vi "algoritmo_3 (1).vi"() -> ()   [LabVIEW 2024]
uses:
  <vilib>/Platform/TimedLoop/XDataNode/timing_clust.ctl
  <vilib>/Platform/TimedLoop/XDataNode/nitl_modes.ctl
  <vilib>/Platform/TimedLoop/XDataNode/wakeup.ctl
  <vilib>/MakerHub/LINX/Public/Peripherals/PWM/PWM Set Duty Cycle 1 Chan.vi
  <vilib>/MakerHub/LINX/Public/Utilities/Open Serial.vi
  <vilib>/MakerHub/LINX/Public/Peripherals/PWM/PWM Set Duty Cycle N Chans.vi
  <vilib>/platform/TimedLoop/XDataNode/XDataNode.xnode
  <vilib>/Platform/TimedLoop/XDataNode/XDNodeRunTimeDep.lvlib
  <vilib>/MakerHub/LINX/LMH-LINX.lvlib
  <vilib>/MakerHub/LINX/Public/Sensors/Distance/Ultrasonic/Ultrasonic.lvlib
  <vilib>/Analysis/NI_AALPro.lvlib
panel:
  in  "MODO":dbl
  in  "Estimacion":dbl(slide) scale=-41.0..41.0
  out "error":dbl
  out "POLO":dbl
  in  "Slide":dbl(slide) scale=-1.0..1.0
  out "PWM":dbl format="%0.2f"
  out "uk":dbl
  in  "Referencia":dbl(slide) scale=10.0..40.0
  out "ESTADO":dbl
  out "MINUTOS":dbl format="%#_2g"
  out "y_estimada":dbl
  out "error de estimacion":dbl
  out "THETA":cdb[](array[numeric])
  out "Waveform Chart":T1(graph)
  in  "stop":bool
  in  "Serial Port":refnum<visa-resource-name>="N/A"
  out "Error Out":errorcluster
  out "Y_Real":fxp<+/-,64,32>
  # "1 PARA CONTROLAR\n0 PARA ESTIMAR"
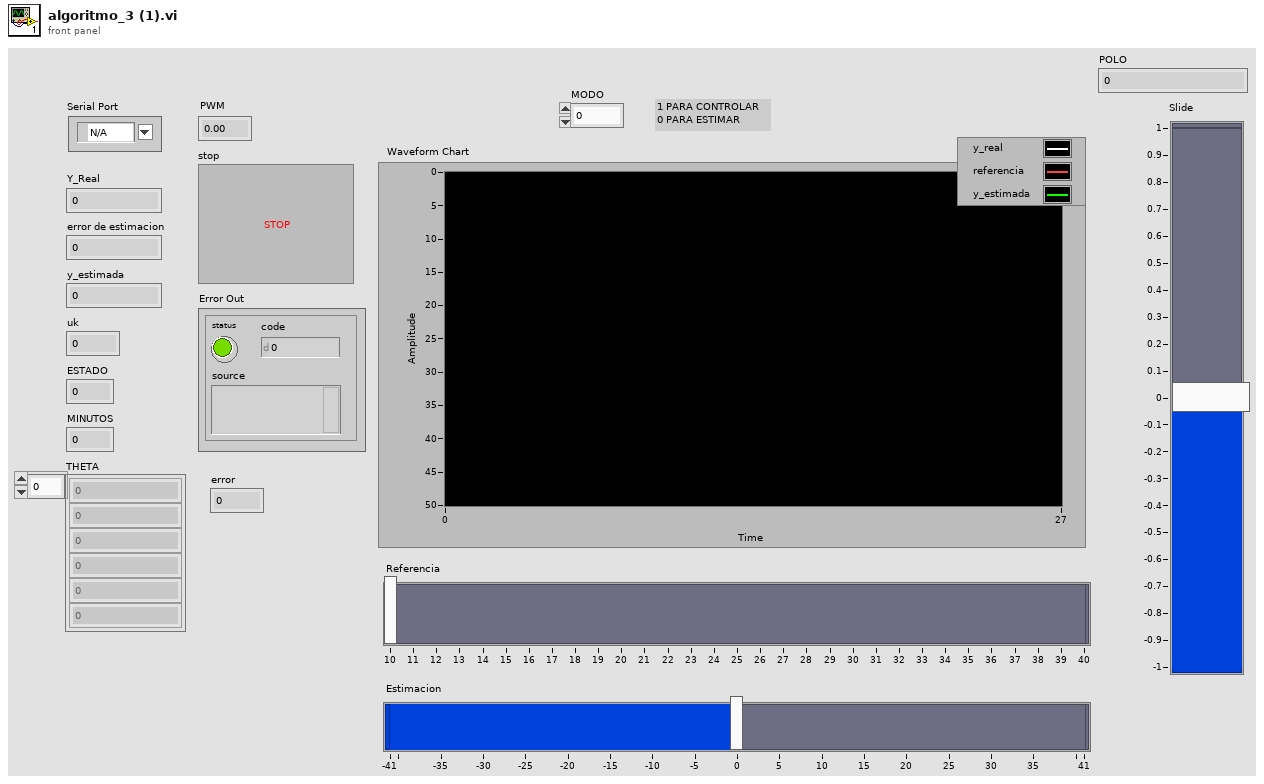
[diagram p1: front panel]
types:
  T1 = cluster{"Centimeters":dbl, "Referencia":dbl, dbl}
  T2 = typedef "LMH-LINX.lvlib/LINX Ref.ctl" = cluster{"IO":T3, "Interface":T4, "LINX Device Config":T5}
  T3 = typedef "LMH-LINX.lvlib/Platform.ctl" = enum16{"Remote", "Local"}
  T4 = typedef "LMH-LINX.lvlib/Interface.ctl" = enum16{"Serial", "TCP"}
  T5 = typedef "LMH-LINX.lvlib/Device.lvlib/LINX Device Config.ctl" = cluster{"Interface":T4, "COM Port":refnum<visa-resource-name>, "TCP Configuration":T6, "Device Family":u8, "Device ID":u8, "Device Name":string, "TCP Ref":refnum<k5>, "Channels":T7}
  T6 = typedef "LMH-LINX.lvlib/Device.lvlib/TCP Config.ctl" = cluster{"IP Address":string, "Port":u16}
  T7 = typedef "LMH-LINX.lvlib/Channels.ctl" = cluster{"DI":u8[], "DO":u8[], "AI":u8[], "AO":u8[], "PWM":u8[], "QE":u8[], "UART":u8[], "I2C 2":u8[], "SPI":u8[], "CAN":u8[], "Servo":u8[], "AI Ref (V)":dbl, "AI Resolution (Bits)":u8, "AO Ref (V)":dbl, "AO Resolution (Bits)":u8}
  T8 = typedef "XDNodeRunTimeDep.lvlib/timing_clust.ctl" = cluster{"Expected End [f-1]":u64, "Actual End [f-1]":u64, "Finished Late? [f-1]":bool, "Expected End [i-1]":u64, "Actual End [i-1]":u64, "Finished Late? [i-1]":bool, "Expected Start [i]":u64, "Actual Start [i]":u64, "Expected Start [f]":u64, "Actual Start [f]":u64, "Source Name":string, "Structure Name":string, "Period":i64, "Deadline":i64, "Offset":i64, "Start":i64, "Priority":i32, "Timeout":i32, "Mode":T9, "Wakeup Reason":T10, "Error":errorcluster, "Source Type":string, "Secondary Source Type":string, "Global End Time":u64, "Global Start Time":u64, "Frame Duration":u64, "Iteration Duration":u64, "Assigned CPU":i32, "I/O Scan Engine Mode":u32}
  T9 = typedef "XDNodeRunTimeDep.lvlib/nitl_modes.ctl" = enum32{"No Change", "Process missed periods, maintain original phase", "Discard missed periods, maintain original phase", "Process missed periods, ignore original phase", "Discard missed periods, ignore original phase"}
  T10 = typedef "XDNodeRunTimeDep.lvlib/wakeup.ctl" = enum32{"Normal", "Aborted", "Asynchronous wakeup", "Timing source error", "Timed loop error", "Timeout"}
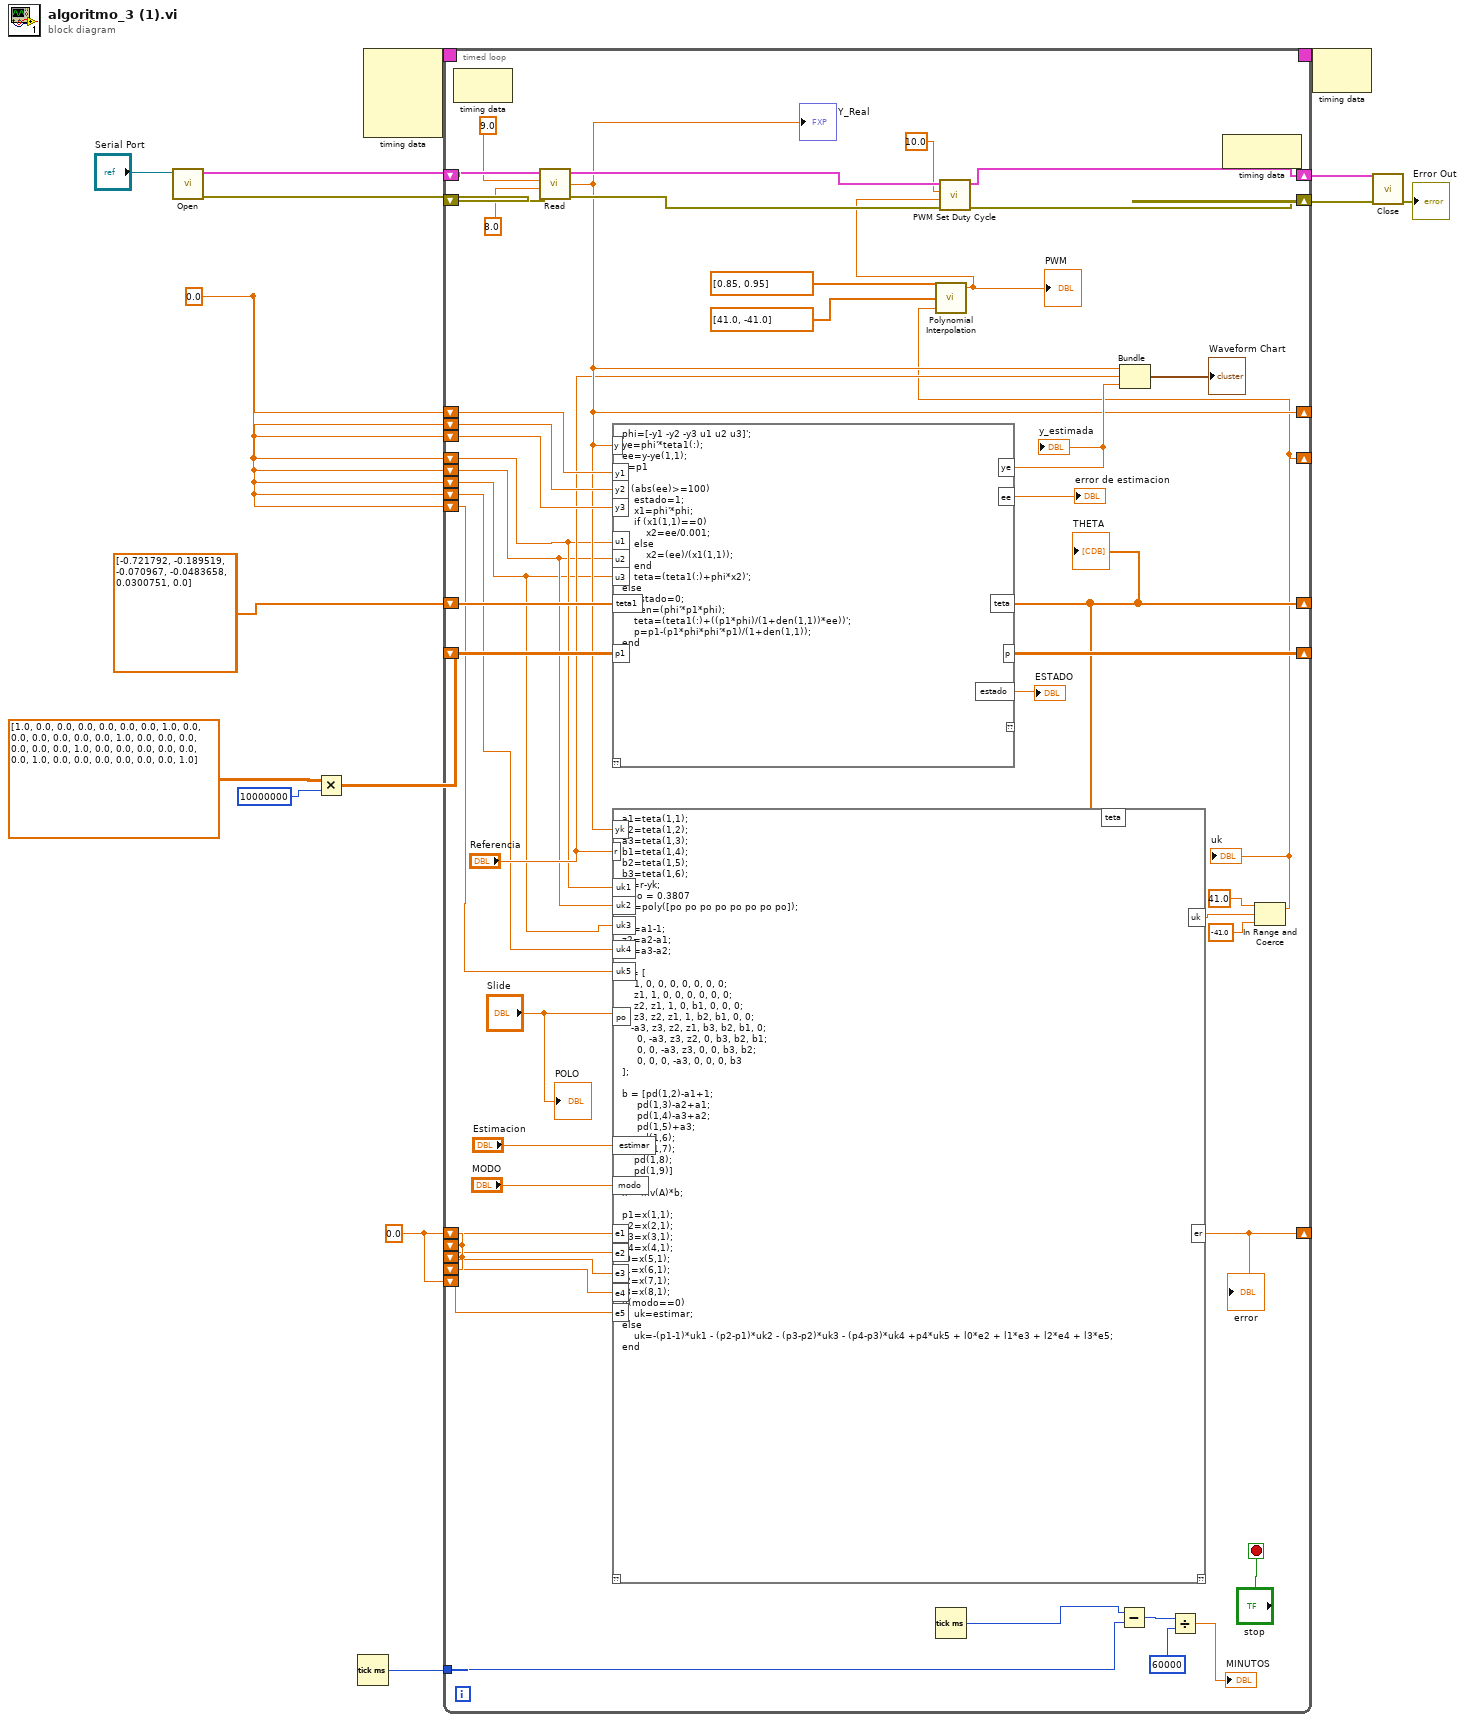
[diagram p0: block diagram]
diagram:
  w2 = 0.0
  (unwired) dbl[] [-0.721792, -0.189519, -0.070967, -0.0483658, 0.0300751, 0.0]
  w1 = 0.0
  n1 = call-poly <vilib>:"Open.vi"("Serial Port"="Serial Port") -> ("Error Out"=w11:errorcluster, "LINX Resource"=w13:T2)  [unwired: 8 in, 1 out]
  n2 = Multiply(x=dbl[][] [[1.0, 0.0, 0.0, 0.0, 0.0, 0.0], [0.0, 1.0, 0.0, 0.0, 0.0, 0.0], [0.0, 0.0, 1.0, 0.0, 0.0, 0.0], [0.0, 0.0, 0.0, 1.0, 0.0, 0.0], [0.0, 0.0, 0.0, 0.0, 1.0, 0.0], [0.0, 0.0, 0.0, 0.0, 0.0, 1.0]], y=10000000) -> (x*y=w5:dbl[][])
  n3 = Tick Count (ms)() -> (millisecond timer value=w4:u32)
  n4 = node-c288() -> (w15:T8)  [unwired: 4 in]
  n5 = timed-loop {
    timing: w15 -> [_]
    timing-out: [_] -> w14
    shift-right: [w52] -> w12
    shift-left: w13 -> [w64]
    shift-right: [w58] -> w10
    shift-left: w11 -> [w63]
    shift-right: [w36] -> _
    shift-left: dbl[] [-1.04495, -0.0852041, 0.125081, 0.000954164, 0.00346055, 0.00317615] -> [w51]
    shift-right: [w35] -> _
    shift-left: w1 -> [w50]
    shift-right: [w30] -> _
    shift-left: w1 -> [w29]
    shift-left: w1 -> [w49]
    shift-left: w1 -> [w48]
    shift-left: w1 -> [w28]
    shift-left: w1 -> [w21]
    shift-right: [w45] -> _
    shift-left: w5 -> [w46]
    tunnel: w4 -> [w41]
    shift-right: [w18] -> _
    shift-left: w2 -> [w26]
    shift-left: w2 -> [w25]
    shift-left: w2 -> [w24]
    shift-left: w2 -> [w23]
    shift-left: w2 -> [w22]
    shift-left: w1 -> [w20]
    shift-left: w1 -> [w19]
    stop <- "stop" stop-if-true
    n6 = node-c288() -> ()  [unwired: 1 in, 1 out]
    n7 = call <vilib>:"Read.vi"("Error In"=w63, "DO Channel"=8.0, "DI Channel"=9.0, "LINX Resource"=w64) -> ("Error Out"=w59:errorcluster, "Centimeters"=w35:dbl, "LINX Resource"=w60:T2)  [unwired: 4 in, 1 out]
    "Y_Real" <- w35
    n8 = script code="phi=[-y1 -y2 -y3 u1 u2 u3]';\nye=phi'*teta1(:);\nee=y-ye(1,1);\np=p1\n\nif (abs(ee)>=100)\n    estado=1;\n    x1=phi'*phi;\n    if (x1(1,1)==0)\n        x2=ee/0.001;\n    else\n        x2=(ee)/(x1(1,1));\n    end\n    teta=(teta1(:)+phi*x2)';\nelse\n    estado=0;\n    den=(phi'*p1*phi);\n    teta=(teta1(:)+((p1*phi)/(1+den(1,1))*ee))';\n    p=p1-(p1*phi*phi'*p1)/(1+den(1,1));\nend"("teta1"=w51, "y1"=w50, "y2"=w49, "y3"=w48, "u1"=w29, "u2"=w28, "u3"=w21, "y"=w35, "p1"=w46) -> ("teta"=w36:dbl[], "p"=w45:dbl[][], "ye"=w44:dbl, "ee"=→"error de estimacion":dbl, "estado"=→"ESTADO":dbl)  [unwired: 1 in, 1 out]
    "THETA" <- w36
    "y_estimada" <- w44
    n9 = script code="a1=teta(1,1);\na2=teta(1,2);\na3=teta(1,3);\nb1=teta(1,4);\nb2=teta(1,5);\nb3=teta(1,6);\ner=r-yk;\n%po = 0.3807\npd=poly([po po po po po po po po]); \n\nz1=a1-1;\nz2=a2-a1;\nz3=a3-a2;\n\nA = [\n    1, 0, 0, 0, 0, 0, 0, 0;\n    z1, 1, 0, 0, 0, 0, 0, 0;\n    z2, z1, 1, 0, b1, 0, 0, 0;\n    z3, z2, z1, 1, b2, b1, 0, 0;\n   -a3, z3, z2, z1, b3, b2, b1, 0;\n     0, -a3, z3, z2, 0, b3, b2, b1;\n     0, 0, -a3, z3, 0, 0, b3, b2;\n     0, 0, 0, -a3, 0, 0, 0, b3\n];\n\nb = [pd(1,2)-a1+1;\n     pd(1,3)-a2+a1;\n     pd(1,4)-a3+a2;\n     pd(1,5)+a3;\n     pd(1,6);\n     pd(1,7);\n    pd(1,8);\n    pd(1,9)]\n\nx = inv(A)*b;\n\np1=x(1,1);\np2=x(2,1);\np3=x(3,1);\np4=x(4,1);\nl0=x(5,1);\nl1=x(6,1);\nl2=x(7,1);\nl3=x(8,1);\nif(modo==0)\n    uk=estimar;\nelse\n    uk=-(p1-1)*uk1 - (p2-p1)*uk2 - (p3-p2)*uk3 - (p4-p3)*uk4 +p4*uk5 + l0*e2 + l1*e3 + l2*e4 + l3*e5;\nend"("teta"=w36, "yk"=w35, "r"="Referencia", "uk1"=w29, "uk2"=w28, "po"="Slide", "e1"=w26, "e2"=w25, "e3"=w24, "e4"=w23, "e5"=w22, "uk3"=w21, "uk4"=w20, "uk5"=w19, "estimar"="Estimacion", "modo"="MODO") -> ("uk"=w31:dbl, "er"=w18:dbl)  [unwired: 1 in, 1 out]
    "error" <- w18
    n10 = Tick Count (ms)() -> (millisecond timer value=w42:u32)
    n11 = Subtract(x=w42, y=w41) -> (x-y=w39:u32)
    n12 = Bundle("Centimeters"=w35, "Referencia"="Referencia", w44) -> (→"Waveform Chart":T1)  [unwired: 1 in]
    n13 = Divide(x=w39, y=u32 60000) -> (x/y=→"MINUTOS":dbl)
    n14 = node-c288() -> ()  [unwired: 1 in, 1 out]
    n15 = In Range and Coerce(upper limit=41.0, x=w31, lower limit=-41.0) -> (coerced(x)=w30:dbl)  [unwired: 1 out]
    "uk" <- w30
    n16 = call <vilib>:"Polynomial Interpolation.vi"("x value"=w30, "X"=dbl[] [41.0, -41.0], "Y"=dbl[] [0.85, 0.95]) -> ("interpolation value"=w54:dbl)  [unwired: 2 out]
    "PWM" <- w54
    n17 = call-poly <vilib>:"PWM Set Duty Cycle.vi"("Error In"=w59, "Duty Cycle (0-1)"=w54, "PWM Channel"=10.0, "LINX Resource"=w60) -> ("Error Out"=w58:errorcluster, "LINX Resource"=w52:T2)  [unwired: 6 in]
    "POLO" <- "Slide"
  }
  n18 = node-c288(w14) -> ()  [unwired: 1 out]
  n19 = call <vilib>:"Close.vi"("Error In"=w10, "LINX Resource"=w12) -> ("Error Out"=→"Error Out":errorcluster)  [unwired: 9 in]
